vi "to SwarmInputArray.vi"(2 "TagArray":refnum<class "Tag.lvclass">[](array[class]), 3 "error in (no error)":errorcluster) -> (7 "SwarmInputArray":T1(array[cluster]), 9 "error IO":errorcluster)   [LabVIEW 2014]
doc: "This VI converts relevant data to swarminputarray to use for swarm method position estimation."
uses:
  Tag.lvclass
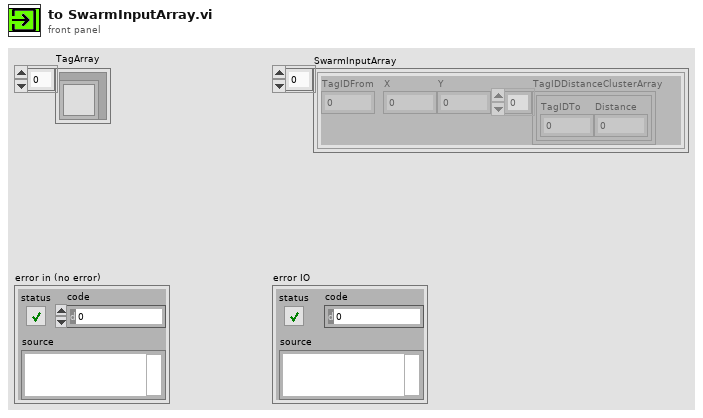
[diagram p1: front panel]
types:
  T1 = cluster{"TagIDFrom":dbl, "X":dbl, "Y":dbl, "TagIDDistanceClusterArray":cluster{"TagIDTo":dbl, "Distance":dbl}[]}[]
  T2 = cluster{"Tag ID":dbl, "TagX":dbl, "TagY":dbl, "TagIDDistanceClusterArray":cluster{"TagIDTo":dbl, "Distance":dbl}[]}
  T3 = cluster{"Tag ID":dbl, "TagX":dbl, "TagY":dbl, "TagIDDistanceClusterArray":cluster{"TagIDTo":dbl, "Distance":dbl}[]}[]
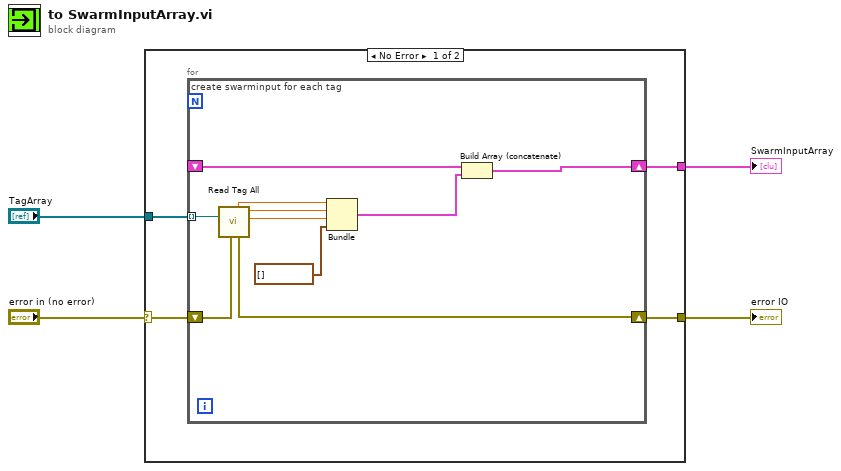
[diagram p0: block diagram]
diagram:
  n1 = case shown="No Error" "error in (no error)" {
    selector: "error in (no error)" -> [w6 w19]
    tunnel: "TagArray" -> [w8 _]
    tunnel: [w7 _] -> w3
    tunnel: [w5 w19] -> w1
    frame No Error {
      n2 = for {
        tunnel: w8 -> [w16] mode=indexing
        shift-right: [w17] -> w7
        shift-left: _ -> [w18]
        shift-right: [w14] -> w5
        shift-left: w6 -> [w15]
        # "create swarminput for each tag"
        n3 = call "Read Tag All.vi"("error in (no error)"=w15, "Tag.lvclass"=w16) -> ("TagY"=w11:dbl, "TagX"=w12:dbl, "error out"=w14:errorcluster, "Tag ID"=w13:dbl)  [unwired: 4 in, 2 out]
        n4 = Bundle("Tag ID"=w13, "TagX"=w12, "TagY"=w11, "TagIDDistanceClusterArray"=cluster{"TagIDTo":dbl, "Distance":dbl}[] []) -> (w9:T2)  [unwired: 1 in]
        n5 = Build Array (concatenate)(w18, w9) -> (w17:T3)
      }
    }
    frame Error {
    }
  }
  "SwarmInputArray" <- w3
  "error IO" <- w1
